vi "Match Pattern.vi"() -> ()   [LabVIEW 2016]
panel:
  out "offset past match":i32
  out "after substring":string
  out "match substring":string
  out "before substring":string
  in  "offset (0)":i32
  in  "regular expression":string
  in  "string":string
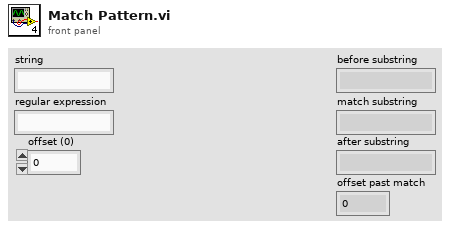
[diagram p1: front panel]
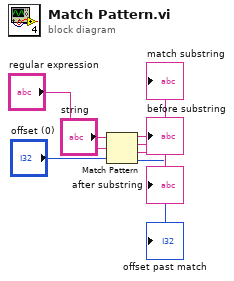
[diagram p0: block diagram]
diagram:
  n1 = Match Pattern(string="string", regular expression="regular expression", offset (0)="offset (0)") -> (before substring=→"before substring":string, match substring=→"match substring":string, after substring=→"after substring":string, offset past match=→"offset past match":i32)
